vi "SavedSettingsRestoreControlValues.vi"(8 "error in (no error)":errorcluster, 10 "SavedValues":cluster{string, string}[](array[cluster]), 11 "ControlTree in":refnum<vi>) -> (0 "error out":errorcluster, 3 "ControlTree out":refnum<vi>)   [LabVIEW 2021]
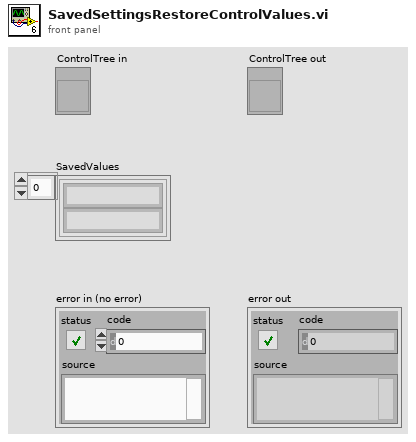
[diagram p1: front panel]
types:
  T1 = cluster{"string array[0]":string, "string array[1]":string, "string array[2]":string}
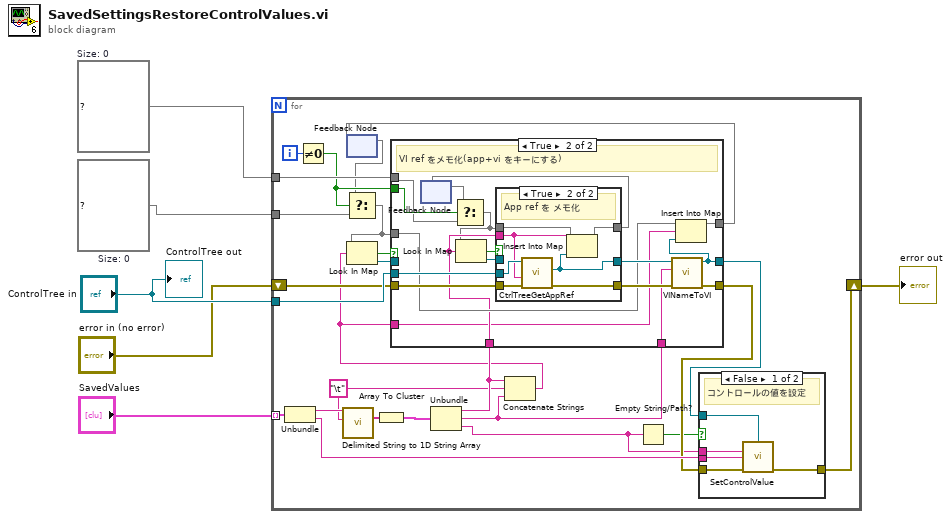
[diagram p0: block diagram]
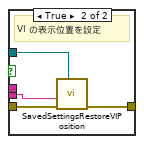
[diagram p4: hidden frame]
diagram:
  w1 = map{string, refnum<vi>} {}  # Size: 0
  w2 = map{string, refnum<vi>} {}  # Size: 0
  n1 = for {
    tunnel: "SavedValues" -> [w31] mode=indexing
    tunnel: "ControlTree in" -> [w27]
    shift-right: [w23] -> w3
    shift-left: "error in (no error)" -> [w25]
    tunnel: w2 -> [w21]
    tunnel: w1 -> [w10]
    i -> [w12]
    w19 = "\t" ("delimiter")
    n2 = Unbundle(w31) -> (w28:string, w26:string)
    n3 = Not Equal To 0?(x=w12) -> (x != 0?=w11:bool)
    n4 = call <vilib>:"Delimited String to 1D String Array.vi"("delimiter"=w19, "delimited string"=w28) -> ("string array"=w30:string[])  [unwired: 9 in]
    n5 = feedback #1() -> (w7:map{string, refnum<vi>})  [unwired: 1 in]
    n6 = Select(t=w7, s=w11, f=w10) -> (s? t:f=w8:map{string, refnum<vi>})
    n7 = Array To Cluster(array=w30) -> (cluster=w29:T1)
    n8 = Unbundle(w29) -> ("string array[0]"=w20:string, "string array[1]"=w15:string, "string array[2]"=w14:string)
    n9 = Concatenate Strings(w20, w19, w15) -> (w13:string)
    n10 = Look In Map(map=w8, key=w13) -> (key not found?=w18:bool, value=w17:refnum<vi>)  [unwired: 1 in]
    n11 = case shown="True" w18 {
      tunnel: w27 -> [_ w52]
      tunnel: w25 -> [w32 w49]
      tunnel: [w32 w46] -> w24
      tunnel: w21 -> [_ w38]
      tunnel: w20 -> [_ w41]
      tunnel: w17 -> [w34 _]
      tunnel: [w34 w42] -> w16
      tunnel: w15 -> [_ w45]
      tunnel: w8 -> [w33 w44]
      tunnel: [w33 w43] -> w9
      tunnel: w13 -> [_ w40]
      tunnel: w11 -> [_ w39]
      frame False {
      }
      frame True {
        # "VI ref をメモ化(app+vi をキーにする)"
        n12 = feedback #2() -> (w36:map{string, refnum<vi>})  [unwired: 1 in]
        n13 = Select(t=w36, s=w39, f=w38) -> (s? t:f=w35:map{string, refnum<vi>})
        n14 = Look In Map(map=w35, key=w41) -> (key not found?=w51:bool, value=w50:refnum<vi>)  [unwired: 1 in]
        n15 = case shown="True" w51 {
          tunnel: w52 -> [_ w57]
          tunnel: [w55 w58] -> w48
          tunnel: w50 -> [w55 _]
          tunnel: w35 -> [w54 w62]
          tunnel: [w54 w61] -> w37
          tunnel: w41 -> [_ w56]
          tunnel: w49 -> [w53 w60]
          tunnel: [w53 w59] -> w47
          frame False {
          }
          frame True {
            # "App ref を メモ化"
            n16 = call "CtrlTreeGetAppRef.vi"("error in (no error)"=w60, "App Tag"=w56, "ControlTree in"=w57) -> ("error out"=w59:errorcluster, "Application out"=w58:refnum<vi>)  [unwired: 5 in, 2 out]
            n17 = Insert Into Map(map in=w62, key=w56, value=w58) -> (map out=w61:map{string, refnum<vi>})  [unwired: 2 out]
          }
        }
        n18 = feedback-in #2(w37) -> ()
        n19 = call "VINameToVI.vi"("error in (no error)"=w47, "vi"=w45, "Application in"=w48) -> ("error out"=w46:errorcluster, "VI out"=w42:refnum<vi>)  [unwired: 7 in]
        n20 = Insert Into Map(map in=w44, key=w40, value=w42) -> (map out=w43:map{string, refnum<vi>})  [unwired: 2 out]
      }
    }
    n21 = feedback-in #1(w9) -> ()
    n22 = Empty String/Path?(string/path=w14) -> (empty?=w22:bool)
    n23 = case shown="False" w22 {
      tunnel: w26 -> [w66 w71]
      tunnel: w24 -> [w65 w69]
      tunnel: [w67 w70] -> w23
      tunnel: w16 -> [w64 w68]
      tunnel: w14 -> [w63 _]
      frame False {
        # "コントロールの値を設定"
        n24 = call "SetControlValue.vi"("vi ref"=w64, "ctrl"=w63, "Value (JSON)"=w66, "error in (no error)"=w65) -> ("error out"=w67:errorcluster)  [unwired: 11 in]
      }
      frame True {
        # "VI の表示位置を設定"
        n25 = call "SavedSettingsRestoreVIPosition.vi"("VI ref"=w68, "error in (no error)"=w69, "Value for VI"=w71) -> ("error out"=w70:errorcluster)  [unwired: 8 in]
      }
    }
  }
  "error out" <- w3
  "ControlTree out" <- "ControlTree in"
